vi "Linix_Get Font Name Array.vi"(8 "error in (no error)":errorcluster) -> (0 "error out":errorcluster, 3 "Font Name Array":string[](array[string]))   [LabVIEW 2021]
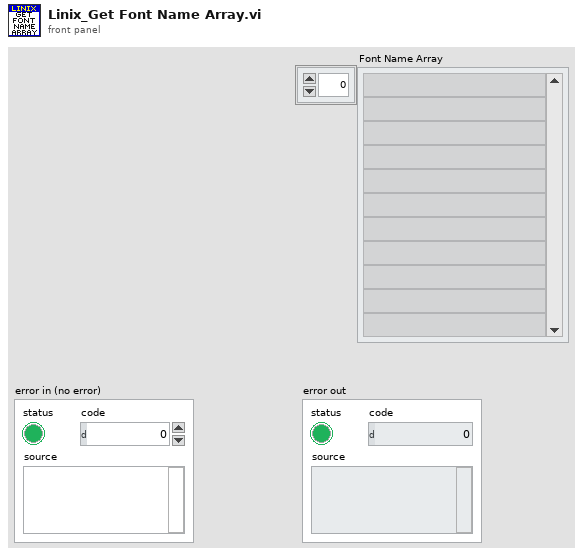
[diagram p1: front panel]
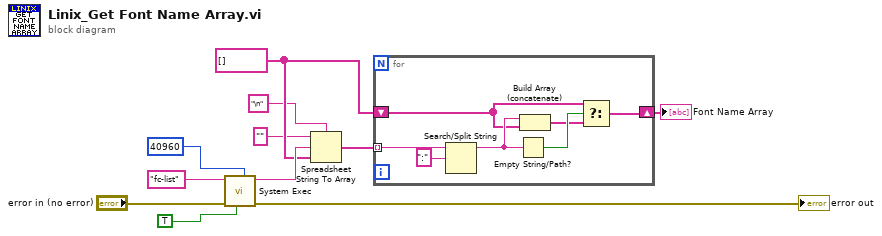
[diagram p0: block diagram]
diagram:
  w7 = string[] []
  n1 = call <vilib>:"System Exec.vi"("expected output size  (4096)"=u32 40960, "run minimized? (F)"=TRUE, "error in (no error)"="error in (no error)", "command line"="fc-list") -> ("error out"=→"error out":errorcluster, "standard output"=w10:string)  [unwired: 3 in, 3 out]
  n2 = Spreadsheet String To Array(delimiter (Tab)="\n", format string="", spreadsheet string=w10, array type (2D Dbl)=w7) -> (array=w6:string[])
  n3 = for {
    tunnel: w6 -> [w18] mode=indexing
    shift-right: [w12] -> w8
    shift-left: w7 -> [w14]
    n4 = Search/Split String(string=w18, search string/char (-)=":") -> (substring before match=w15:string)  [unwired: 3 out]
    n5 = Empty String/Path?(string/path=w15) -> (empty?=w16:bool)
    n6 = Build Array (concatenate)(w15, w14) -> (w13:string[])
    n7 = Select(t=w14, s=w16, f=w13) -> (s? t:f=w12:string[])
  }
  "Font Name Array" <- w8
